vi "Initialize.vi"(8 "error in":errorcluster, 10 "parameters":variant, 11 "node in":refnum<class "ScaleAndLimitModule editor node.lvclass">) -> (0 "error out":errorcluster, 2 "summary":T2[](array[typedef]), 3 "data value reference":T1)   [LabVIEW 2017, in "ScaleAndLimitModule editor node.lvclass"]
doc: "Initializes the data of a node to its default state.\nThe object is not created inside of this VI, because it is created from a File depending on user selection."
uses:
  ScaleAndLimitModule editor node.lvclass
  C:/Program Files (x86)/National Instruments/LabVIEW 2017/vi.lib/NI/Configuration Framework/Node/NISE_CEF_Node.lvclass
  <vilib>/NI/Configuration Framework/Node/Summary.ctl
  <vilib>/NI/Configuration Framework/Node/NodeRef.ctl
  <vilib>/NI/Configuration Framework/Node/NISE_CEF_Node.lvclass
  module/configuration/ScaleAndLimitModule configuration.lvclass
  C:/Program Files (x86)/National Instruments/LabVIEW 2017/vi.lib/NI/Configuration Framework/serializable configuration/NISE_CEF_serializable configuration.lvclass
  <vilib>/NI/PowerElectronicsControl/ScaleAndLimit/Interface/Configuration.ctl
  module/configuration/ScaleAndLimitModule configuration.lvclass/ScaleAndLimitModule configuration.ctl
  module/configuration/Write ScaleAndLimitConfig.vi
  <vilib>/NI/DCAF/Tag Editor Core/control module/editor node/control module editor.lvclass
  <vilib>/NI/Configuration Framework/serializable configuration/NISE_CEF_serializable configuration.lvclass
  <vilib>/NI/PowerElectronicsControl/ScaleAndLimit/Interface/ScaleAndLimitInterface.lvlib
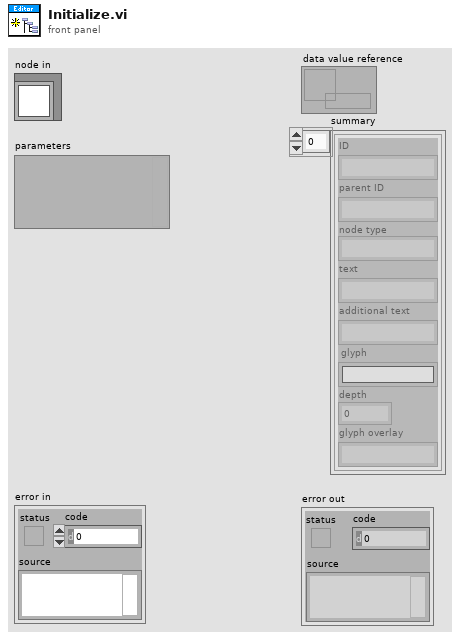
[diagram p1: front panel]
types:
  T1 = typedef "NISE_CEF_Node.lvclass/NodeRef.ctl" = refnum<data-value>
  T2 = typedef "NISE_CEF_Node.lvclass/Summary.ctl" = cluster{"ID":string, "parent ID":string, "node type":string, "text":string, "additional text":string, "glyph":string, "depth":i32, "glyph overlay":string}
  T3 = typedef "ScaleAndLimitInterface.lvlib/Configuration.ctl" = cluster{"Name":string, "M":dbl, "B":i16, "HighLimit":dbl, "LowLimit":dbl, "LimitsEnabled":bool}
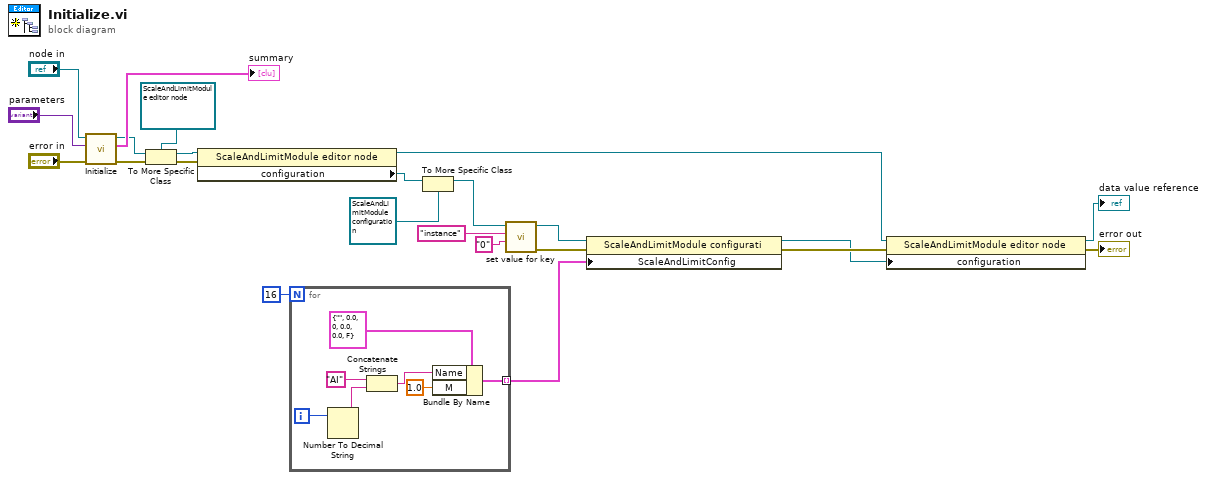
[diagram p0: block diagram]
diagram:
  n1 = call-parent "Initialize.vi"("error in"="error in", "parameters"="parameters", "node in"="node in") -> ("error out"=w15:errorcluster, "summary"=→"summary":T2[], "data value reference"=w16:T1)  [unwired: 6 in]
  n2 = To More Specific Class(target class=refnum<data-value> refnum ("data value reference"), reference=w16, error in=w15) -> (specific class reference=w14:refnum<data-value>, error out=w17:errorcluster)
  n3 = property class="ScaleAndLimitModule editor node"(reference=w14, error in=w17) -> (reference out=w9:refnum<data-value>, "configuration"=w10:refnum<class "NISE_CEF_serializable configuration.lvclass">)  [unwired: 1 out]
  n4 = for {
    N: 16 -> [_]
    tunnel: [w24] -> w1 mode=indexing
    i -> [w29]
    n5 = Number To Decimal String(number=w29) -> (decimal integer string=w27:string)  [unwired: 1 in]
    n6 = Concatenate Strings("AI", w27) -> (w26:string)
    n7 = Bundle By Name(cluster=T3 {"Name"="", "M"=0.0, "B"=0, "HighLimit"=0.0, "LowLimit"=0.0, "LimitsEnabled"=FALSE} ("Configuration"), "Name"=w26, "M"=1.0) -> (w24:T3)
  }
  n8 = To More Specific Class(target class=refnum<class "ScaleAndLimitModule configuration.lvclass"> refnum ("ScaleAndLimitModule configuration"), reference=w10) -> (specific class reference=w11:refnum<class "ScaleAndLimitModule configuration.lvclass">)  [unwired: 1 in, 1 out]
  n9 = call-dynamic "set value for key.vi"("value"="0", "key"="instance", "fixed channel configuration in"=w11) -> ("error out"=w5:errorcluster, "fixed channel configuration out"=w6:refnum<class "ScaleAndLimitModule configuration.lvclass">)  [unwired: 7 in]
  n10 = property class="ScaleAndLimitModule configurati"(reference=w6, error in=w5, "ScaleAndLimitConfig"=w1) -> (reference out=w3:refnum<class "ScaleAndLimitModule configuration.lvclass">, error out=w4:errorcluster)
  n11 = property class="ScaleAndLimitModule editor node"(reference=w9, error in=w4, "configuration"=w3) -> (reference out=→"data value reference":refnum<data-value>, error out=→"error out":errorcluster)
